vi "Revision Query Core.vi"(8 "error in (no error)":errorcluster, 11 "BNT_ULx-MCSV in":refnum<class "BNT_ULx-MCSV.lvclass">) -> (0 "error out":errorcluster, 1 "Firmware Revision":string, 2 "Driver Revision":string, 3 "BNT_ULx-MCSV out":refnum<class "BNT_ULx-MCSV.lvclass">)   [LabVIEW 2020, in "BNT_ULx.lvlib" / "BNT_ULx-MCSV.lvclass"]
uses:
  BNT_ULx-MCSV.lvclass
  CSPP_Core/Actors/CSPP_DeviceActor/CSPP_DeviceActor.lvclass
  BNT_ULx-MCSV.lvclass/BNT_ULx-MCSV.ctl
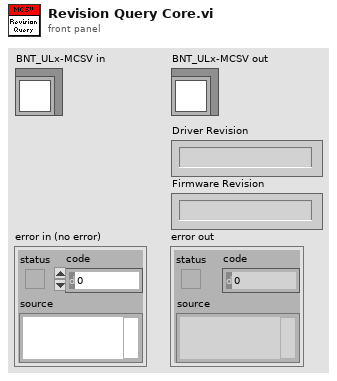
[diagram p1: front panel]
types:
  T1 = cluster{"Major":u16, "Minor":u16, "Fix":u16, "Build":u16}
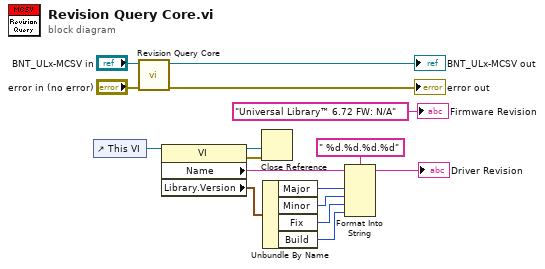
[diagram p0: block diagram]
diagram:
  n1 = control-ref of="This VI"() -> (w12:refnum<vi>)
  n2 = call-parent "Revision Query Core.vi"("error in (no error)"="error in (no error)", "CSPP_DeviceActor in"="BNT_ULx-MCSV in") -> ("error out"=→"error out":errorcluster, "CSPP_DeviceActor out"=→"BNT_ULx-MCSV out":refnum<class "BNT_ULx-MCSV.lvclass">)  [unwired: 6 in, 2 out]
  n3 = property class="VI"(reference=w12) -> (reference out=w10:refnum<vi>, error out=w11:errorcluster, "Name"=w7:string, "Library.Version"=w9:T1)  [unwired: 1 in]
  n4 = Close Reference(reference=w10, error in (no error)=w11) -> ()  [unwired: 1 out]
  n5 = Unbundle By Name(w9) -> ("Major"=w6:u16, "Minor"=w5:u16, "Fix"=w4:u16, "Build"=w3:u16)
  n6 = Format Into String(format string=" %d.%d.%d.%d" ("Driver Revision"), initial string=w7, w6, w5, w4, w3) -> (resulting string=→"Driver Revision":string)  [unwired: 1 in, 1 out]
  "Firmware Revision" <- "Universal Library™ 6.72 FW: N/A" ("Firmware Revision")
